vi "Is var in acceptable range.vi"(1 "Variable":dbl, 2 "Acceptable plus minus":dbl) -> (0 "Acceptable":bool)   [LabVIEW 2019]
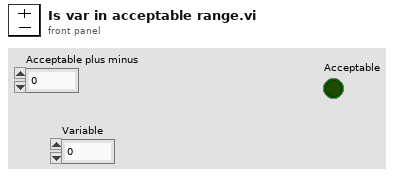
[diagram p1: front panel]
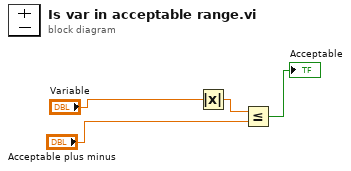
[diagram p0: block diagram]
diagram:
  n1 = Absolute Value(x="Variable") -> (abs(x)=w3:dbl)
  n2 = Less Or Equal?(x=w3, y="Acceptable plus minus") -> (x <= y?=→"Acceptable":bool)
